vi "Initialize Ring Control.vi"(8 "error in (no error)":errorcluster, 9 "Values":string[][](array[string]), 10 "Caption.Text":string, 11 "Ring":refnum<vi>) -> (0 "error out":errorcluster, 3 "Ring out":refnum<vi>)   [LabVIEW 2013, in "Ring Workspace Object.lvlib"]
uses:
  Ring Workspace Object.lvlib
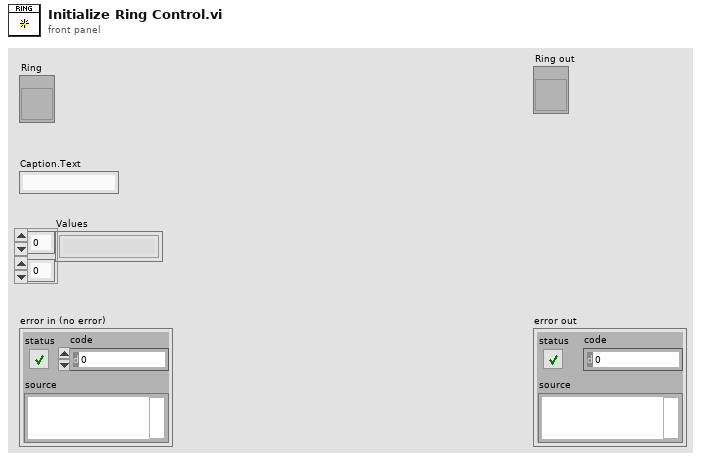
[diagram p1: front panel]
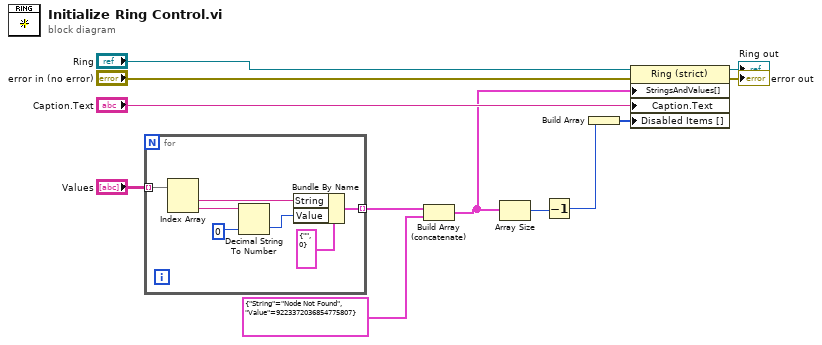
[diagram p0: block diagram]
diagram:
  n1 = for {
    tunnel: "Values" -> [w19] mode=indexing
    tunnel: [w13] -> w6 mode=indexing
    n2 = Index Array(array=w19) -> (element #1=w17:string, element #2=w16:string)  [unwired: 2 in]
    n3 = Decimal String To Number(string=w16, default (0L)=i64 0 ("Value")) -> (number=w14:i64)  [unwired: 1 in, 1 out]
    n4 = Bundle By Name(cluster=cluster{"String":string, "Value":i64} {"String"="", "Value"=0}, "String"=w17, "Value"=w14) -> (w13:cluster{"String":string, "Value":i64})
  }
  n5 = Build Array (concatenate)(w6, cluster{"String":string, "Value":i64} {"String"="Node Not Found", "Value"=9223372036854775807}) -> (w4:cluster{"String":string, "Value":i64}[])
  n6 = Array Size(array=w4) -> (size(s)=w3:i32)
  n7 = Decrement(x=w3) -> (x-1=w2:i32)
  n8 = Build Array(w2) -> (w1:i32[])
  n9 = property class="Ring (strict)"(reference="Ring", error in="error in (no error)", "StringsAndValues[]"=w4, "Caption.Text"="Caption.Text", "Disabled Items []"=w1) -> (reference out=→"Ring out":refnum<vi>, error out=→"error out":errorcluster)
